vi "Main Dialog.vi"(8 "error in (no error)":errorcluster, 11 "New Class Dialog in":refnum<class "New Class Dialog.lvclass">) -> (0 "error out":errorcluster, 3 "New Class Dialog out":refnum<class "New Class Dialog.lvclass">)   [LabVIEW 2020, in "New Class Dialog.lvclass"]
uses:
  New Class Dialog.lvclass
panel:
  in  "Parent Class":string(tree)
  in  "Process Name":string
  in  "Save to Folder":path
  in  "Commit":bool
  in  "Cancel":bool
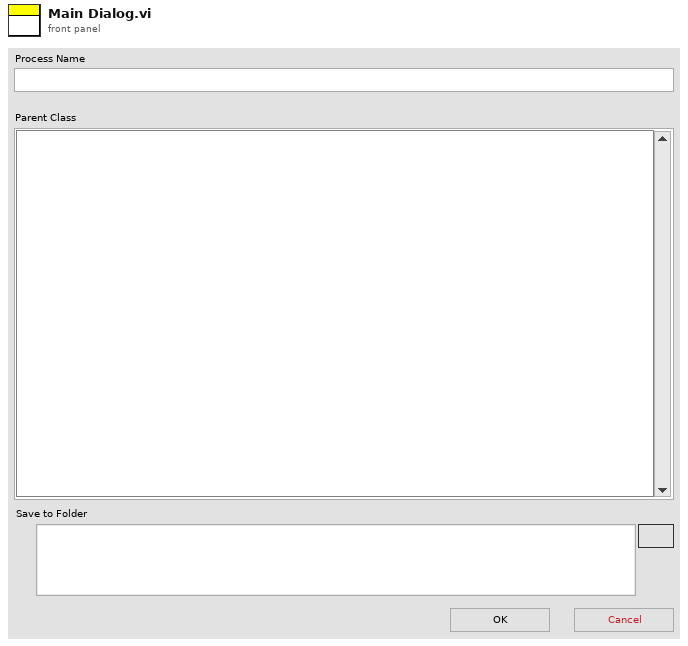
[diagram p1: front panel]
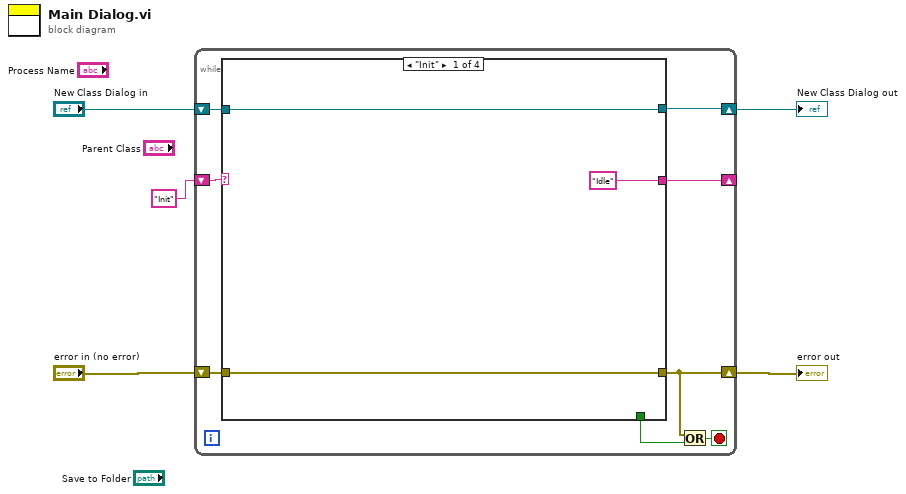
[diagram p0: block diagram]
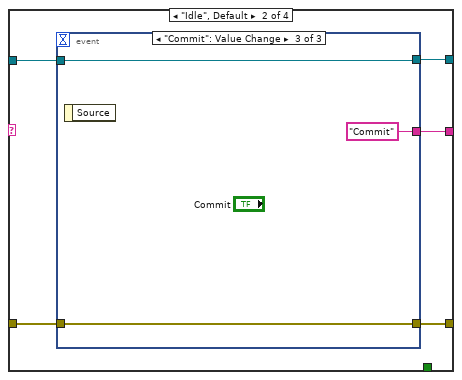
[diagram p2: hidden frame]
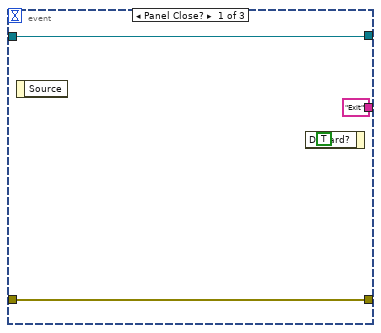
[diagram p3: hidden frame]
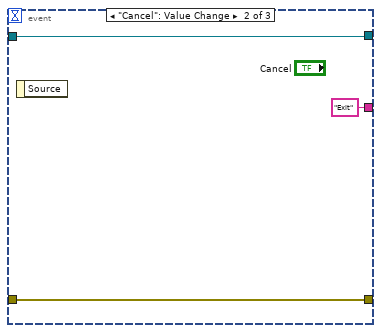
[diagram p4: hidden frame]
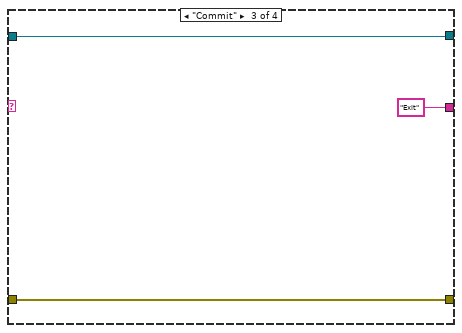
[diagram p5: hidden frame]
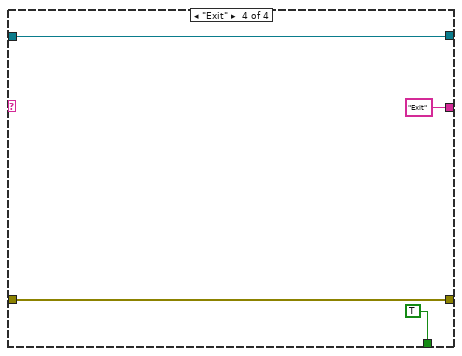
[diagram p6: hidden frame]
diagram:
  n1 = while {
    shift-right: [w10] -> w3
    shift-left: "New Class Dialog in" -> [w11]
    shift-right: [w6] -> w2
    shift-left: "error in (no error)" -> [w12]
    shift-right: [w9] -> _
    shift-left: "Init" -> [w13]
    stop <- w7 stop-if-true
    n2 = case shown="\"Init\"" w13 {
      tunnel: [w16 w21 w34 w37] -> w6
      tunnel: w12 -> [w16 w20 w34 w37]
      tunnel: w11 -> [w15 w19 w33 w38]
      tunnel: [w15 w18 w33 w38] -> w10
      tunnel: ["Idle" w17 "Exit" "Exit"] -> w9
      tunnel: [_ _ _ TRUE] -> w8
      frame "Init" {
      }
      frame "Idle", Default {
        n3 = event shown="[2] \"Commit\": Value Change" {
          selector: _ -> [_ _ _]
          dyn-events: _ -> [_ _ _]
          timeout: _ -> [_ _ _]
          tunnel: [w25 w27 w31] -> w21
          tunnel: w20 -> [w25 w27 w31]
          tunnel: w19 -> [w24 w28 w30]
          tunnel: [w24 w28 w30] -> w18
          tunnel: ["Exit" "Exit" "Commit"] -> w17
          event Panel Close? {
            n4 = event-data() -> ()  [unwired: 1 in, 1 out]
            n5 = event-data("Discard?"=TRUE) -> ()  [unwired: 1 in, 1 out]
          }
          event "Cancel": Value Change {
            n6 = event-data() -> ()  [unwired: 1 in, 1 out]
          }
          event "Commit": Value Change {
            n7 = event-data() -> ()  [unwired: 1 in, 1 out]
          }
        }
      }
      frame "Commit" {
      }
      frame "Exit" {
      }
    }
    n8 = Or(x=w6, y=w8) -> (x .or. y?=w7:bool)
  }
  "error out" <- w2
  "New Class Dialog out" <- w3
